vi "Connect to stage.vi"(8 "error in (no error)":errorcluster, 10 "Hardware State":T2, 11 "Hardware Configuration":T1={"VISA resource name"="", "Timeout (3sec)"=3000}) -> (0 "error out":errorcluster, 2 "Hardware State Out":T2, 3 "Hardware Configuration Out":T1={"VISA resource name"="", "Timeout (3sec)"=3000})   [LabVIEW 2015, in "XYZStage.lvlib"]
uses:
  XYZStage.lvlib
  XYZStage State.ctl
  XYZStage Loop State.ctl
  XYZStage Configuration.ctl
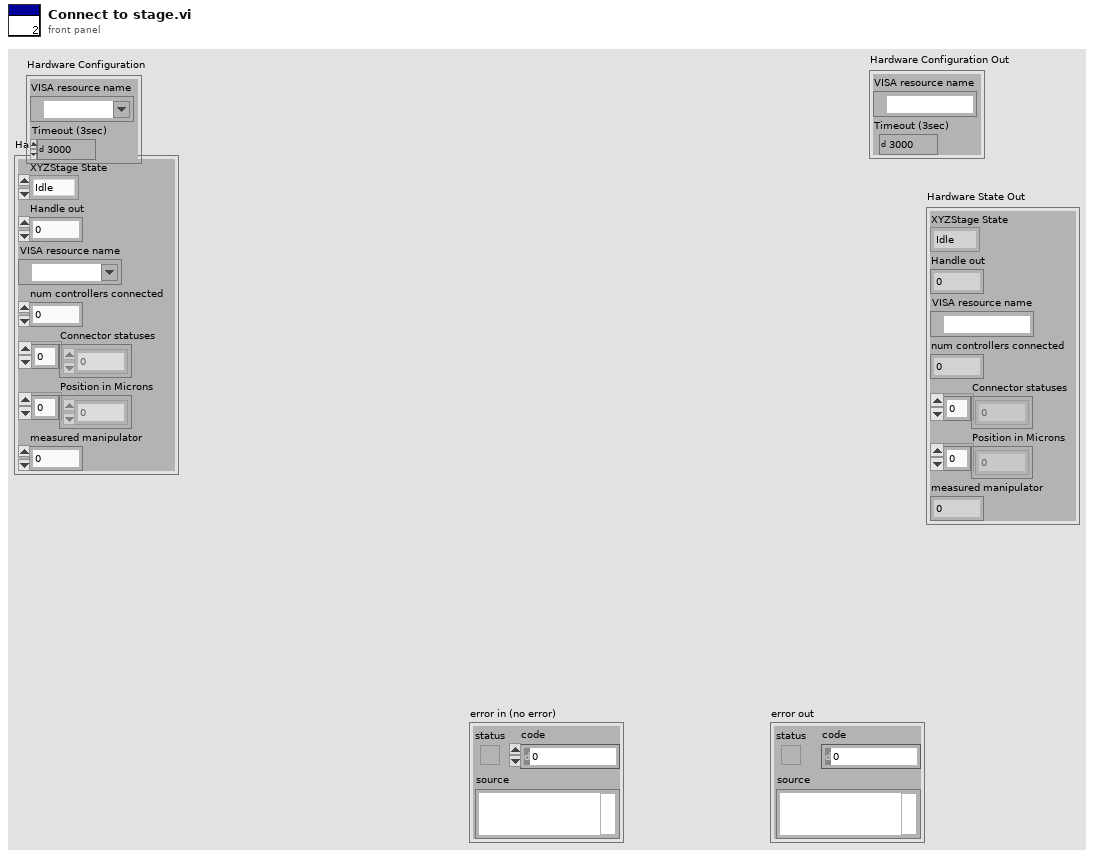
[diagram p1: front panel]
types:
  T1 = typedef "XYZStage.lvlib/XYZStage Configuration.ctl" = cluster{"VISA resource name":refnum<visa-resource-name>, "Timeout (3sec)":u32}
  T2 = typedef "XYZStage.lvlib/XYZStage State.ctl" = cluster{"XYZStage State":T3, "Handle out":u32, "VISA resource name":refnum<visa-resource-name>, "num controllers connected":u8, "Connector statuses":u8[], "Position in Microns":dbl[], "measured manipulator":u8}
  T3 = typedef "XYZStage.lvlib/XYZStage Loop State.ctl" = enum16{"Idle", "Connected", "Moving"}
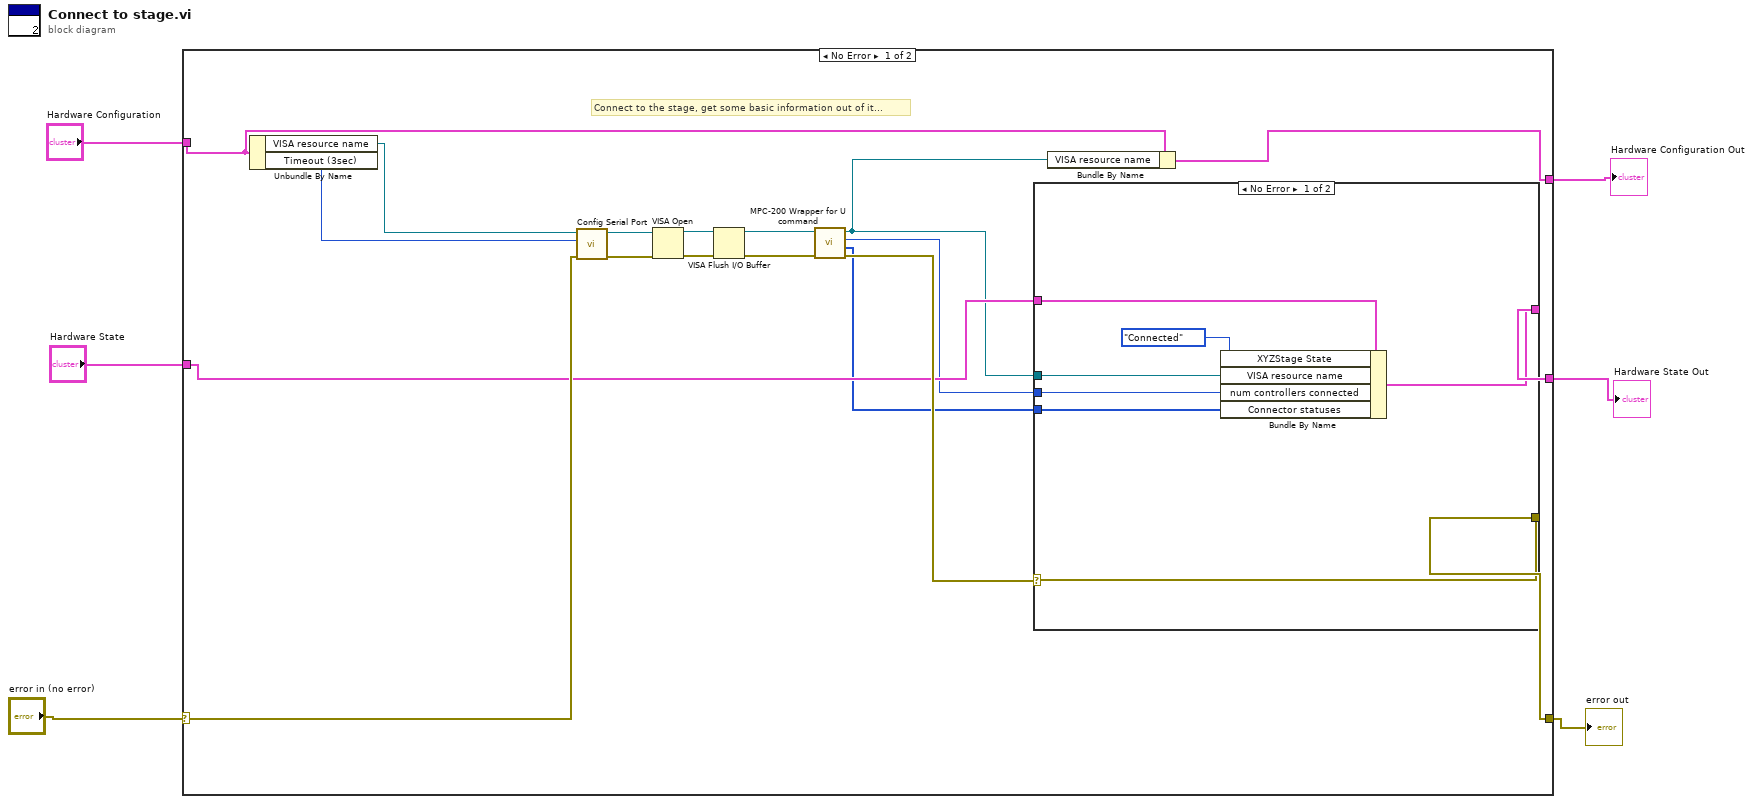
[diagram p0: block diagram]
diagram:
  n1 = case shown="No Error" "error in (no error)" {
    selector: "error in (no error)" -> [w22 w36]
    tunnel: [w10 w36] -> w5
    tunnel: [w14 w35] -> w4
    tunnel: "Hardware Configuration" -> [w15 w35]
    tunnel: [w11 w34] -> w2
    tunnel: "Hardware State" -> [w12 w34]
    frame No Error {
      # "Connect to the stage, get some basic information out of it..."
      n2 = Unbundle By Name(w15) -> ("VISA resource name"=w24:refnum<visa-resource-name>, "Timeout (3sec)"=w23:u32)
      n3 = call "Config Serial Port.vi"("error in (no error)"=w22, "Timeout (3sec)"=w23, "VISA resource name"=w24) -> ("error out"=w20:errorcluster, "VISA resource name out"=w21:refnum<visa-resource-name>)  [unwired: 7 in]
      n4 = VISA Open(error in (no error)=w20, VISA resource name=w21) -> (VISA resource name=w18:refnum<visa-resource-name>, error out=w19:errorcluster)  [unwired: 3 in]
      n5 = VISA Flush I/O Buffer(VISA resource name=w18, error in (no error)=w19) -> (VISA resource name out=w16:refnum<visa-resource-name>, error out=w17:errorcluster)  [unwired: 1 in]
      n6 = call "MPC-200 Wrapper for U command.vi"("error in (no error)"=w17, "VISA resource name in"=w16) -> ("error out"=w13:errorcluster, "Connector statuses"=w7:u8[], "num controllers connected"=w8:u8, "VISA resource name out"=w9:refnum<visa-resource-name>)  [unwired: 6 in]
      n7 = case shown="No Error" w13 {
        selector: w13 -> [w28 w32]
        tunnel: w12 -> [w31 w33]
        tunnel: [w30 w33] -> w11
        tunnel: [w28 w32] -> w10
        tunnel: w9 -> [w27 _]
        tunnel: w8 -> [w26 _]
        tunnel: w7 -> [w25 _]
        frame No Error {
          n8 = Bundle By Name(cluster=w31, "XYZStage State"=XYZStage_Loop_State."Connected", "VISA resource name"=w27, "num controllers connected"=w26, "Connector statuses"=w25) -> (w30:T2)
        }
        frame Error {
        }
      }
      n9 = Bundle By Name(cluster=w15, "VISA resource name"=w9) -> (w14:T1)
    }
    frame Error {
    }
  }
  "error out" <- w5
  "Hardware State Out" <- w2
  "Hardware Configuration Out" <- w4
